vi "Disabled.vi"(7 "Robot Mode":T2, 10 "Match Info":T1={"Autonomous Elapsed Seconds"=0.0, "TeleOp Elapsed Seconds"=0.0, "Disabled Elapsed Seconds"=0.0, "Visited Autonomous"=FALSE, "Visited TeleOp"=FALSE, "Visited Disabled"=FALSE, "Autonomous Settings"={"Autonomous Style"=enum."Independent", "VI Refnum"=refnum}}, 11 "Call Context":T3) -> ()   [LabVIEW 2013]
doc: "This VI is called each time a disabled packet is received from the DS. It is often used to prepare for the next robot mode, to calibrate sensors, etc."
uses:
  <vilib>/Rock Robotics/WPI/DriverStation/WPI_DriverStationDerivedRobotMode.ctl
  <vilib>/Rock Robotics/WPI/DriverStation/WPI_DriverStationRobotMode2.ctl
  <vilib>/Rock Robotics/WPI/DriverStation/WPI_DriverStationMatch Info.ctl
  QueueAction.ctl
  TankDriveAction.ctl
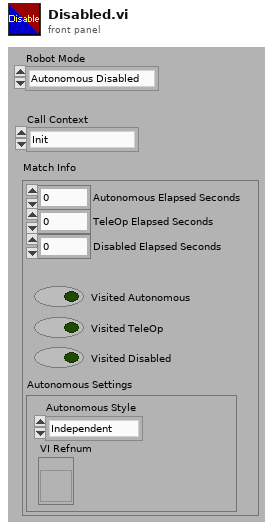
[diagram p1: front panel]
types:
  T1 = typedef "WPI_DriverStationMatch Info.ctl" = cluster{"Autonomous Elapsed Seconds":dbl, "TeleOp Elapsed Seconds":dbl, "Disabled Elapsed Seconds":dbl, "Visited Autonomous":bool, "Visited TeleOp":bool, "Visited Disabled":bool, "Autonomous Settings":cluster{"Autonomous Style":enum16{"Iterative", "Independent"}, "VI Refnum":refnum<vi>}}
  T2 = typedef "WPI_DriverStationRobotMode2.ctl" = enum16{"Autonomous Disabled", "Autonomous Enabled", "Teleop Disabled", "Teleop Enabled", "Timeout", "Finish", "Test Disabled", "Test Enabled"}
  T3 = typedef "WPI_DriverStationDerivedRobotMode.ctl" = enum16{"Init", "Execute", "Stop"}
  T4 = typedef "TankDriveAction.ctl" = enum16{"Init", "LinearDrive", "SetValue", "Disable"}
  T5 = typedef "QueueAction.ctl" = enum16{"Init", "SetValue", "Disable"}
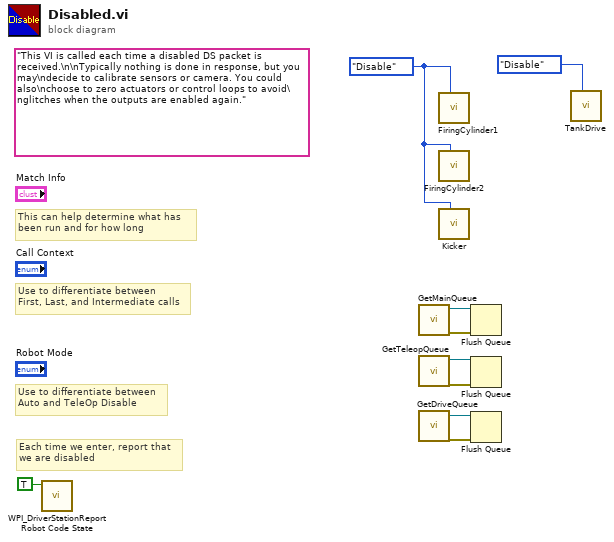
[diagram p0: block diagram]
diagram:
  w8 = QueueAction."Disable" ("Action")
  (unwired) "This VI is called each time a disabled DS packet is received.\n\nTypically nothing is done in response, but you may\ndecide to calibrate sensors or camera. You could also\nchoose to zero actuators or control loops to avoid\nglitches when the outputs are enabled again."
  # "Each time we enter, report that\nwe are disabled"
  # "Use to differentiate between\nFirst, Last, and Intermediate calls"
  # "This can help determine what has\nbeen run and for how long"
  # "Use to differentiate between\nAuto and TeleOp Disable"
  n1 = call <vilib>:"WPI_DriverStationReport Robot Code State.vi"("Disabled"=TRUE ("Autonomous")) -> ()  [unwired: 10 in, 1 out]
  n2 = call "GetMainQueue.vi"() -> ("error out"=w6:errorcluster, "queue out"=w5:refnum<queue>)  [unwired: 10 in]
  n3 = call "GetTeleopQueue.vi"() -> ("error out"=w4:errorcluster, "queue out"=w3:refnum<queue>)  [unwired: 10 in]
  n4 = call "GetDriveQueue.vi"() -> ("error out"=w1:errorcluster, "queue out"=w2:refnum<queue>)  [unwired: 10 in]
  n5 = call "FiringCylinder1.vi"("Action"=w8) -> ()  [unwired: 10 in, 1 out]
  n6 = call "FiringCylinder2.vi"("Action"=w8) -> ()  [unwired: 10 in, 1 out]
  n7 = call "Kicker.vi"("Action"=w8) -> ()  [unwired: 10 in, 1 out]
  n8 = Flush Queue(queue=w5, error in (no error)=w6) -> ()  [unwired: 3 out]
  n9 = Flush Queue(queue=w3, error in (no error)=w4) -> ()  [unwired: 3 out]
  n10 = Flush Queue(queue=w2, error in (no error)=w1) -> ()  [unwired: 3 out]
  n11 = call "TankDrive.vi"("DriveAction"=TankDriveAction."Disable") -> ()  [unwired: 9 in, 2 out]
